vi "REACTOR_CHANGE.vi"(9 "error in (no error)":errorcluster, 10 "Change":T1) -> (1 "error out":errorcluster, 2 "Change?":T1)   [LabVIEW 2017]
uses:
  REACTOR_CHANGE.ctl
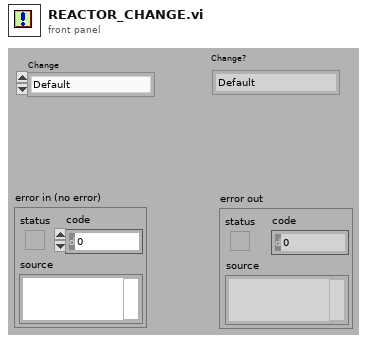
[diagram p1: front panel]
types:
  T1 = typedef "REACTOR_CHANGE.ctl" = enum16{"Default", "Continue", "Change Alicats", "Change Valve", "Change Calor", "Change Frio"}
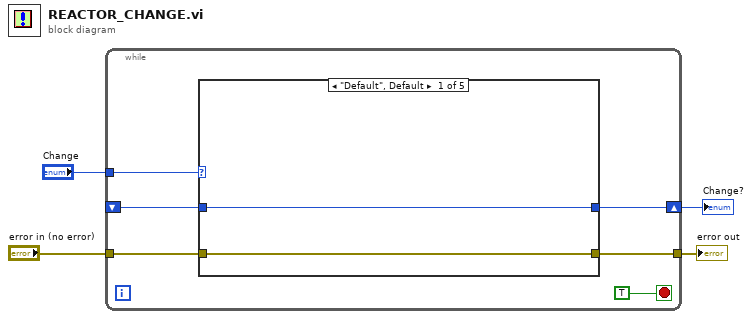
[diagram p0: block diagram]
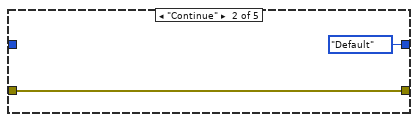
[diagram p2: hidden frame]
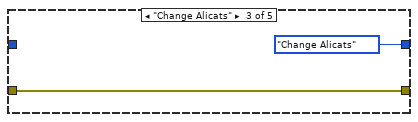
[diagram p3: hidden frame]
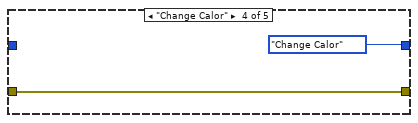
[diagram p4: hidden frame]
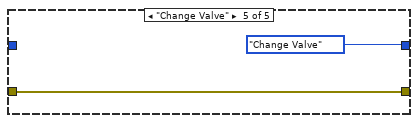
[diagram p5: hidden frame]
diagram:
  n1 = while {
    tunnel: "Change" -> [w10]
    shift-right: [w8] -> w3
    shift-left: _ -> [w7]
    tunnel: "error in (no error)" -> [w6]
    tunnel: [w5] -> w1
    stop <- TRUE stop-if-true
    n2 = case shown="\"Default\", Default" w10 {
      tunnel: [w12 REACTOR_CHANGE."Default" ("Change 2") REACTOR_CHANGE."Change Alicats" ("Change") REACTOR_CHANGE."Change Calor" ("Change") REACTOR_CHANGE."Change Valve" ("Change")] -> w8
      tunnel: w7 -> [w12 _ _ _ _]
      tunnel: w6 -> [w11 w14 w16 w18 w20]
      tunnel: [w11 w14 w16 w18 w20] -> w5
      frame "Default", Default {
      }
      frame "Continue" {
      }
      frame "Change Alicats" {
      }
      frame "Change Calor" {
      }
      frame "Change Valve" {
      }
    }
  }
  "Change?" <- w3
  "error out" <- w1
